vi "getScanValues.vi"(8 "error in (no error)":errorcluster, 11 "ScanCreator in":refnum<class "ScanCreator.lvclass">) -> (0 "error out":errorcluster, 1 "stop":dbl, 2 "start":dbl, 3 "ScanCreator out":refnum<class "ScanCreator.lvclass">, 4 "step":i16, 5 "increment":dbl)   [LabVIEW 2011, in "Views.lvlib" / "ScriptEditor.lvlib" / "ScanCreator.lvclass"]
uses:
  ScanCreator.lvclass
  ScanCreator.lvclass/ScanCreator.ctl
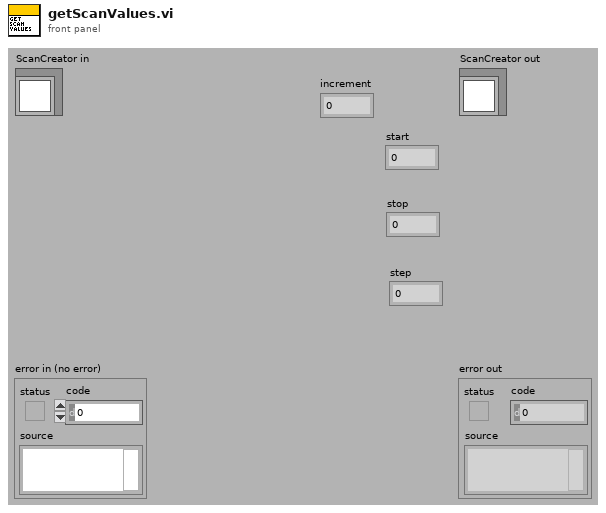
[diagram p1: front panel]
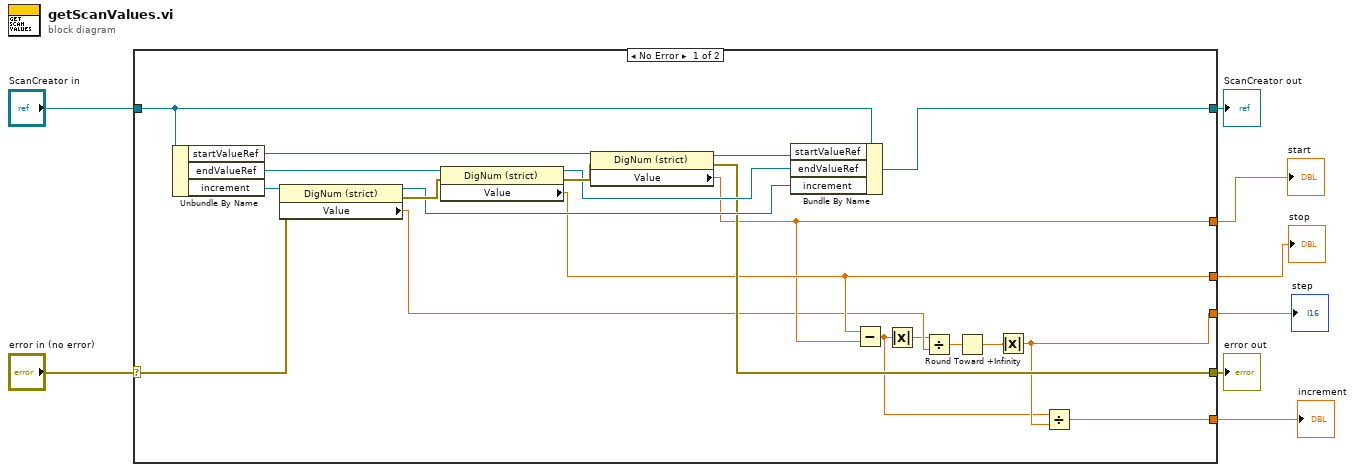
[diagram p0: block diagram]
diagram:
  n1 = case shown="No Error" "error in (no error)" {
    selector: "error in (no error)" -> [w24 w31]
    tunnel: [w20 w31] -> w7
    tunnel: [w18 w30] -> w5
    tunnel: "ScanCreator in" -> [w19 w30]
    tunnel: [w11 _] -> w4
    tunnel: [w16 _] -> w3
    tunnel: [w15 _] -> w2
    tunnel: [w9 _] -> w1
    frame No Error {
      n2 = Unbundle By Name(w19) -> ("startValueRef"=w27:refnum<vi>, "endValueRef"=w28:refnum<vi>, "increment"=w29:refnum<vi>)
      n3 = property class="DigNum (strict)"(reference=w29, error in=w24) -> (reference out=w21:refnum<vi>, error out=w25:errorcluster, "Value"=w14:dbl)
      n4 = property class="DigNum (strict)"(reference=w28, error in=w25) -> (reference out=w22:refnum<vi>, error out=w26:errorcluster, "Value"=w16:dbl)
      n5 = property class="DigNum (strict)"(reference=w27, error in=w26) -> (reference out=w23:refnum<vi>, error out=w20:errorcluster, "Value"=w15:dbl)
      n6 = Bundle By Name(cluster=w19, "startValueRef"=w23, "endValueRef"=w22, "increment"=w21) -> (w18:refnum<class "ScanCreator.lvclass">)
      n7 = Subtract(x=w16, y=w15) -> (x-y=w10:dbl)
      n8 = Absolute Value(x=w10) -> (abs(x)=w12:dbl)
      n9 = Divide(x=w12, y=w14) -> (x/y=w17:dbl)
      n10 = Round Toward +Infinity(x=w17) -> (ceil(x): smallest int >= x=w13:dbl)
      n11 = Absolute Value(x=w13) -> (abs(x)=w11:dbl)
      n12 = Divide(x=w10, y=w11) -> (x/y=w9:dbl)
    }
    frame Error {
    }
  }
  "error out" <- w7
  "ScanCreator out" <- w5
  "start" <- w2
  "stop" <- w3
  "step" <- w4
  "increment" <- w1
